vi "Gate-Delay.vi"(4 "Delay (tick)":i64, 6 "Gated (tick)":i64, 7 "Analog input":bool, 8 "addcounter":i64, 9 "adshift2":bool, 10 "adshift1":bool, 11 "Refnum in":refnum<k21>="ConnectorA/DIO0") -> (0 "adcounter'":i64, 1 "adshift2'":bool, 2 "adshift1'":bool, 3 "signal out":bool)   [LabVIEW 2018]
uses:
  <vilib>/rvi/eio/common/nirviEmuTemplateMethod_errors.vi
  <vilib>/eio/EIONode/EIONode.xnode
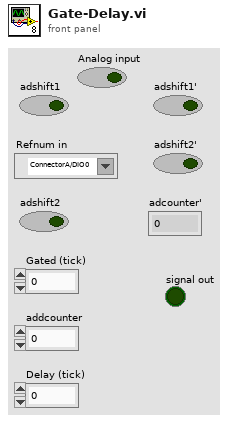
[diagram p1: front panel]
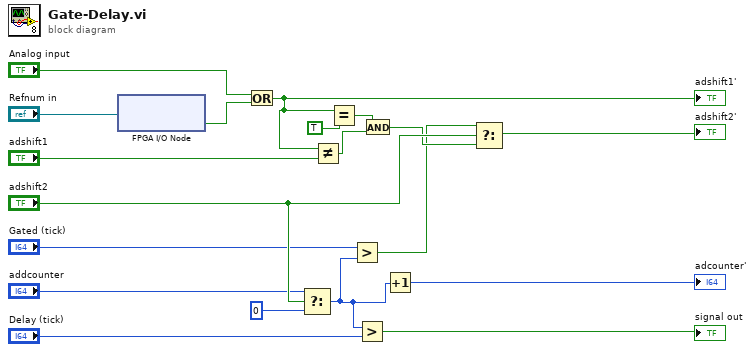
[diagram p0: block diagram]
diagram:
  n1 = xnode "FPGA I/O Node"("FPGA I/O In"="Refnum in") -> ("I/O Item"=w2:bool)  [unwired: 1 out]
  n2 = Or(x="Analog input", y=w2) -> (x .or. y?=w3:bool)
  "adshift1'" <- w3
  n3 = Select(t="addcounter", s="adshift2", f=i64 0) -> (s? t:f=w12:i64)
  n4 = Not Equal?(x=w3, y="adshift1") -> (x != y?=w15:bool)
  n5 = Equal?(x=w3, y=TRUE) -> (x = y?=w14:bool)
  n6 = Greater?(x="Gated (tick)", y=w12) -> (0:w10:bool)
  n7 = Greater?(x=w12, y="Delay (tick)") -> (0:→"signal out":bool)
  n8 = And(x=w14, y=w15) -> (x .and. y?=w17:bool)
  n9 = Increment(x=w12) -> (x+1=→"adcounter'":i64)
  n10 = Select(t=w10, s="adshift2", f=w17) -> (s? t:f=→"adshift2'":bool)
